vi "Agilent_Get_ScanList.vi"(6 "Building 35?":bool, 9 "Number of Elements":i32=16) -> (0 "Scan List Array":string[](array[string]), 1 "Scanlist":string, 3 "Temporary Labels 2":string[](array[string])=["TC Evap1 - IN", "TC Evap2", "TC Evap3", "TC Evap4", "TC Evap5 - OUT", "TC Xtra 1", "TC Xtra 2", "TC Xtra 3", "TC Xtra 4", "TC Dry/W bulb 1", "TC Dry/W bulb 2", "TC Dry/W bulb 3", "TC Dry/W bulb 4", "TC Tsuction", "TC Tdis", "TC Tret", "TC Controls 1", "TC Controls 2", "TC Controls 3", "TC Controls 4", "TC Controls 5", "TC Shadow T1", "TC Shadow T2", "TC Shadow T3", "TC Shadow T4", "TC Shadow T5", "TC Shadow T6", "TC Xtra 5", "TC Xtra 6", "TC Xtra 7", "TC Xtra 8", "TC Xtra 9", "TC Cond1 - IN", "TC Cond2", "TC Cond3", "TC Cond4", "TC Cond5", "TC Cond6", "TC Cond7", "TC Cond8", "TC Cond9", "TC Cond10", "TC Cond11", "TC Cond12 - OUT", "NC", "NC", "NC", "NC"])   [LabVIEW 2013]
panel:
  in  "Temporary Labels":string[](array[string])=["TC Evap1 - IN", "TC Evap2", "TC Evap3", "TC Evap4", "TC Evap5 - OUT", "TC Xtra 1", "TC Xtra 2", "TC Xtra 3", "TC Xtra 4", "TC Dry/W bulb 1", "TC Dry/W bulb 2", "TC Dry/W bulb 3", "TC Dry/W bulb 4", "TC Tsuction", "TC Tdis", "TC Tret", "TC Controls 1", "TC Controls 2", "TC Controls 3", "TC Controls 4", "TC Controls 5", "TC Shadow T1", "TC Shadow T2", "TC Shadow T3", "TC Shadow T4", "TC Shadow T5", "TC Shadow T6", "TC Xtra 5", "TC Xtra 6", "TC Xtra 7", "TC Xtra 8", "TC Xtra 9", "TC Cond1 - IN", "TC Cond2", "TC Cond3", "TC Cond4", "TC Cond5", "TC Cond6", "TC Cond7", "TC Cond8", "TC Cond9", "TC Cond10", "TC Cond11", "TC Cond12 - OUT", "NC", "NC", "NC", "NC"]
  in  "Agilent Scan List":string="101,102,103,104,105,106,107,108,109,110,111,112,113,114,115,116"
  # "Takes as input the number of elements to be scanned on the Agilent."
  # "Assumes that the elements are wired in order."
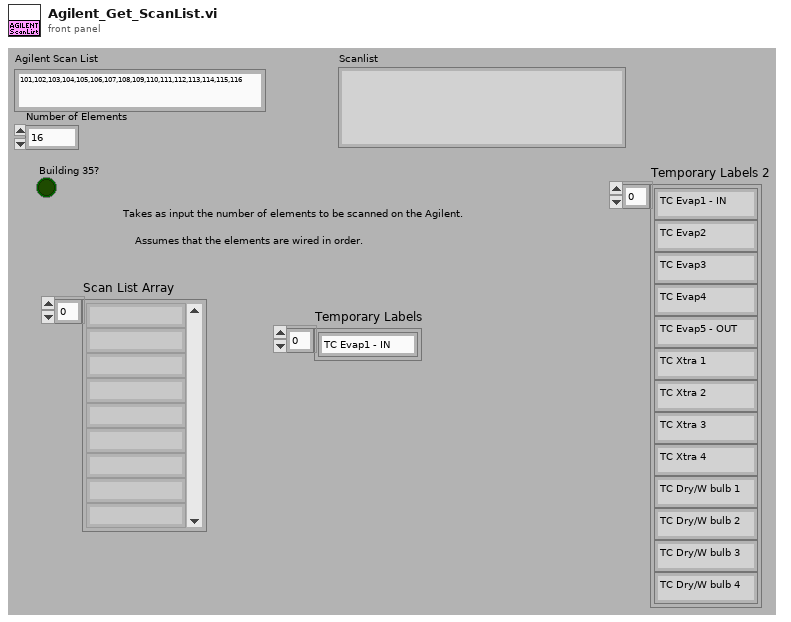
[diagram p1: front panel]
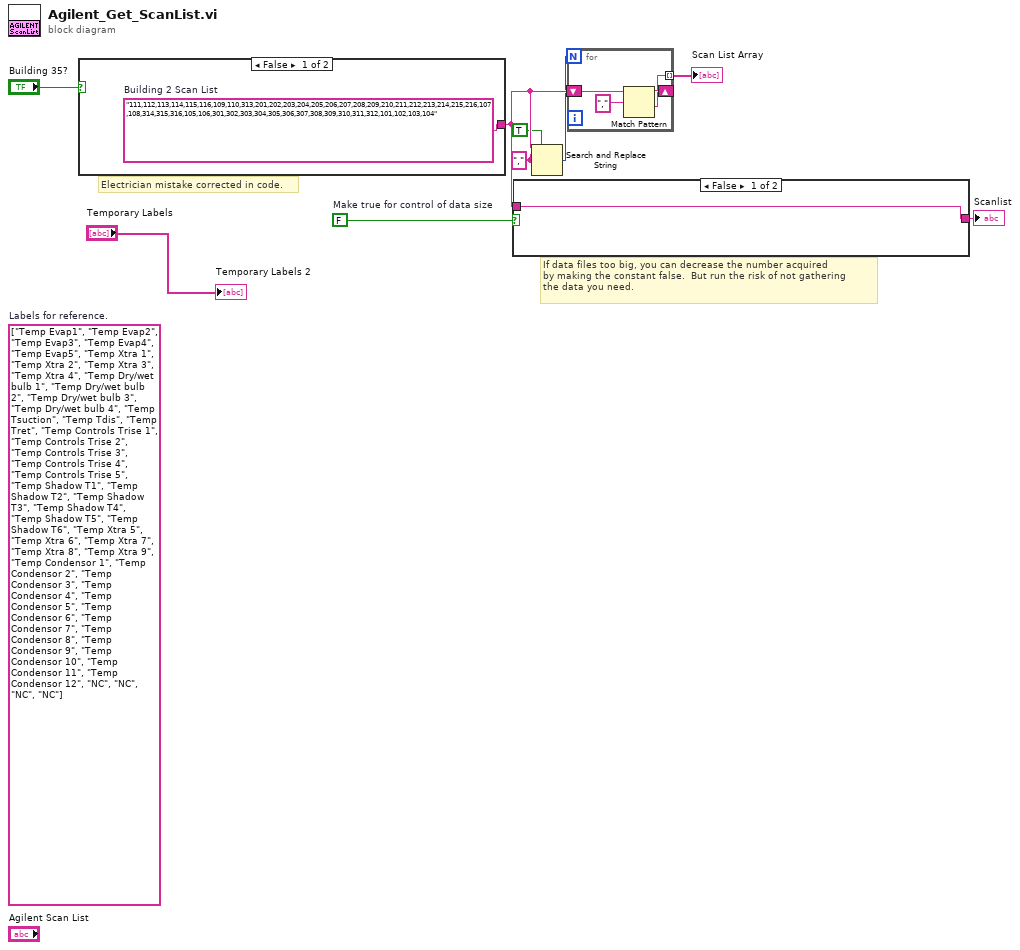
[diagram p0: block diagram]
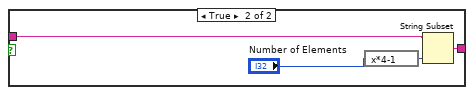
[diagram p2: hidden frame]
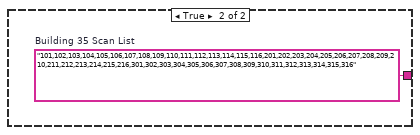
[diagram p3: hidden frame]
diagram:
  w2 = "," ("search string")
  (unwired) string[] ["Temp Evap1", "Temp Evap2", "Temp Evap3", "Temp Evap4", "Temp Evap5", "Temp Xtra 1", "Temp Xtra 2", "Temp Xtra 3", "Temp Xtra 4", "Temp Dry/wet bulb 1", "Temp Dry/wet bulb 2", "Temp Dry/wet bulb 3", "Temp Dry/wet bulb 4", "Temp Tsuction", "Temp Tdis", "Temp Tret", "Temp Controls Trise 1", "Temp Controls Trise 2", "Temp Controls Trise 3", "Temp Controls Trise 4", "Temp Controls Trise 5", "Temp Shadow T1", "Temp Shadow T2", "Temp Shadow T3", "Temp Shadow T4", "Temp Shadow T5", "Temp Shadow T6", "Temp Xtra 5", "Temp Xtra 6", "Temp Xtra 7", "Temp Xtra 8", "Temp Xtra 9", "Temp Condensor 1", "Temp Condensor 2", "Temp Condensor 3", "Temp Condensor 4", "Temp Condensor 5", "Temp Condensor 6", "Temp Condensor 7", "Temp Condensor 8", "Temp Condensor 9", "Temp Condensor 10", "Temp Condensor 11", "Temp Condensor 12", "NC", "NC", "NC", "NC"]  # Labels for reference.
  w7 = FALSE  # Make true for control of data size
  # "If data files too big, you can decrease the number acquired\nby making the constant false.  But run the risk of not gathering \nthe data you need."
  # "Electrician mistake corrected in code."
  n1 = case shown="False" "Building 35?" {
    tunnel: [w10 w11] -> w5
    frame False {
      w10 = "111,112,113,114,115,116,109,110,313,201,202,203,204,205,206,207,208,209,210,211,212,213,214,215,216,107,108,314,315,316,105,106,301,302,303,304,305,306,307,308,309,310,311,312,101,102,103,104"  # Building 2 Scan List
    }
    frame True {
      w11 = "101,102,103,104,105,106,107,108,109,110,111,112,113,114,115,116,201,202,203,204,205,206,207,208,209,210,211,212,213,214,215,216,301,302,303,304,305,306,307,308,309,310,311,312,313,314,315,316"  # Building 35 Scan List
    }
  }
  n2 = case shown="False" w7 {
    tunnel: [w12 w14] -> w9
    tunnel: w5 -> [w12 w13]
    frame False {
    }
    frame True {
      n3 = expression code="x*4-1"("Number of Elements") -> (w15:i32)
      n4 = String Subset(string=w13, length (rest)=w15) -> (substring=w14:string)  [unwired: 1 in]
    }
  }
  "Scanlist" <- w9
  n5 = Search and Replace String(replace all?=TRUE ("replace all? (F)"), input string=w5, search string=w2, replace string=w2) -> (number of replacements=w3:i32)  [unwired: 4 in, 3 out]
  n6 = for {
    N: w3 -> [_]
    tunnel: [w18] -> w6 mode=indexing
    shift-right: [w17] -> _
    shift-left: w5 -> [w20]
    n7 = Match Pattern(string=w20, regular expression=",") -> (before substring=w18:string, after substring=w17:string)  [unwired: 1 in, 2 out]
  }
  "Scan List Array" <- w6
  "Temporary Labels 2" <- "Temporary Labels"
